vi "Generate_WayPoints_Hopping_IT_Surface.vi"(11 "Input Cluster":T2={"Scan Rate (um/s)"=15.0, "X Start"=15.0, "X End"=15.0, "Y Start"=15.0, "Y End"=15.0, " Z Start"=15.0, "HoppingDistance"=1.0, "V"=15.0, "Z End"=15.0, "Approach Rate Hopping (um/s)"=15.0, "Retrack Rate (um/s)"=15.0, "V 1"=15.0, "HoldTime IT/s"=15.0, "HoldTime Bulk Pre IT/s 2"=15.0, "HoldTime Bulk IT Post/s"=15.0, "V2"=0.0, "HoldTime IT 2/s"=15.0}) -> (0 "output cluster":T1, 3 "WaitTimeScaler":u64)   [LabVIEW 2023]
uses:
  TypeDefs/WayPointCluster.ctl
  TypeDefsControls/Time.ctl
  User_Vi/Settings.vi
panel:
  in  "WayPointCluster":T1
  out "Y  P":dbl
  out "X  P":dbl
  out "HoppingDistanceX":dbl
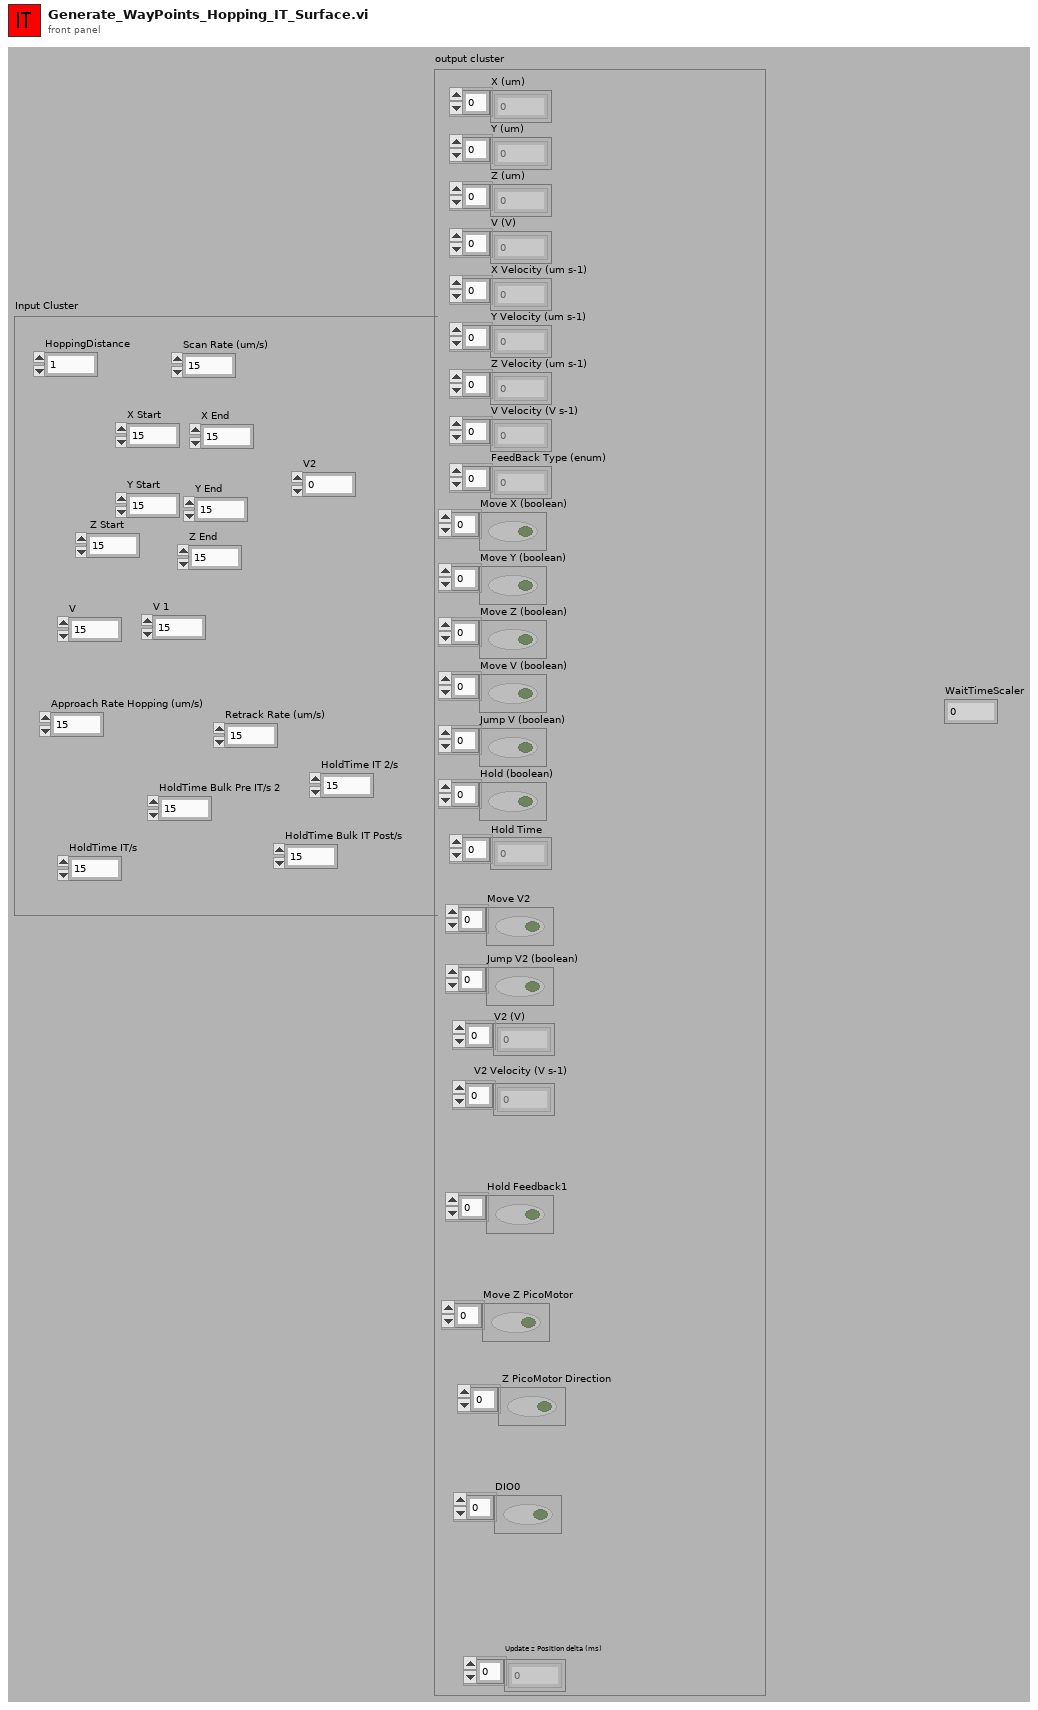
[diagram p1: front panel]
types:
  T1 = typedef "WayPointCluster.ctl" = cluster{"X (um)":dbl[], "Y (um)":dbl[], "Z (um)":dbl[], "V (V)":dbl[], "X Velocity (um s-1)":dbl[], "Y Velocity (um s-1)":dbl[], "Z Velocity (um s-1)":dbl[], "V Velocity (V s-1)":dbl[], "FeedBack Type (enum)":u16[], "Move X (boolean)":bool[], "Move Y (boolean)":bool[], "Move Z (boolean)":bool[], "Move V (boolean)":bool[], "Jump V (boolean)":bool[], "Hold (boolean)":bool[], "Hold Time":u32[], "V2 (V)":dbl[], "Move V2":bool[], "V2 Velocity (V s-1)":dbl[], "Jump V2 (boolean)":bool[], "Update z Position delta (ms)":i16[], "Hold Feedback1":bool[], "Move Z PicoMotor":bool[], " Z PicoMotor Direction":bool[], "DIO0":bool[]}
  T2 = cluster{"Scan Rate (um/s)":dbl, "X Start":dbl, "X End":dbl, "Y Start":dbl, "Y End":dbl, " Z Start":dbl, "HoppingDistance":dbl, "V":dbl, "Z End":dbl, "Approach Rate Hopping (um/s)":dbl, "Retrack Rate (um/s)":dbl, "V 1":dbl, "HoldTime IT/s":dbl, "HoldTime Bulk Pre IT/s 2":dbl, "HoldTime Bulk IT Post/s":dbl, "V2":dbl, "HoldTime IT 2/s":dbl}
  T3 = typedef "Time.ctl" = dbl
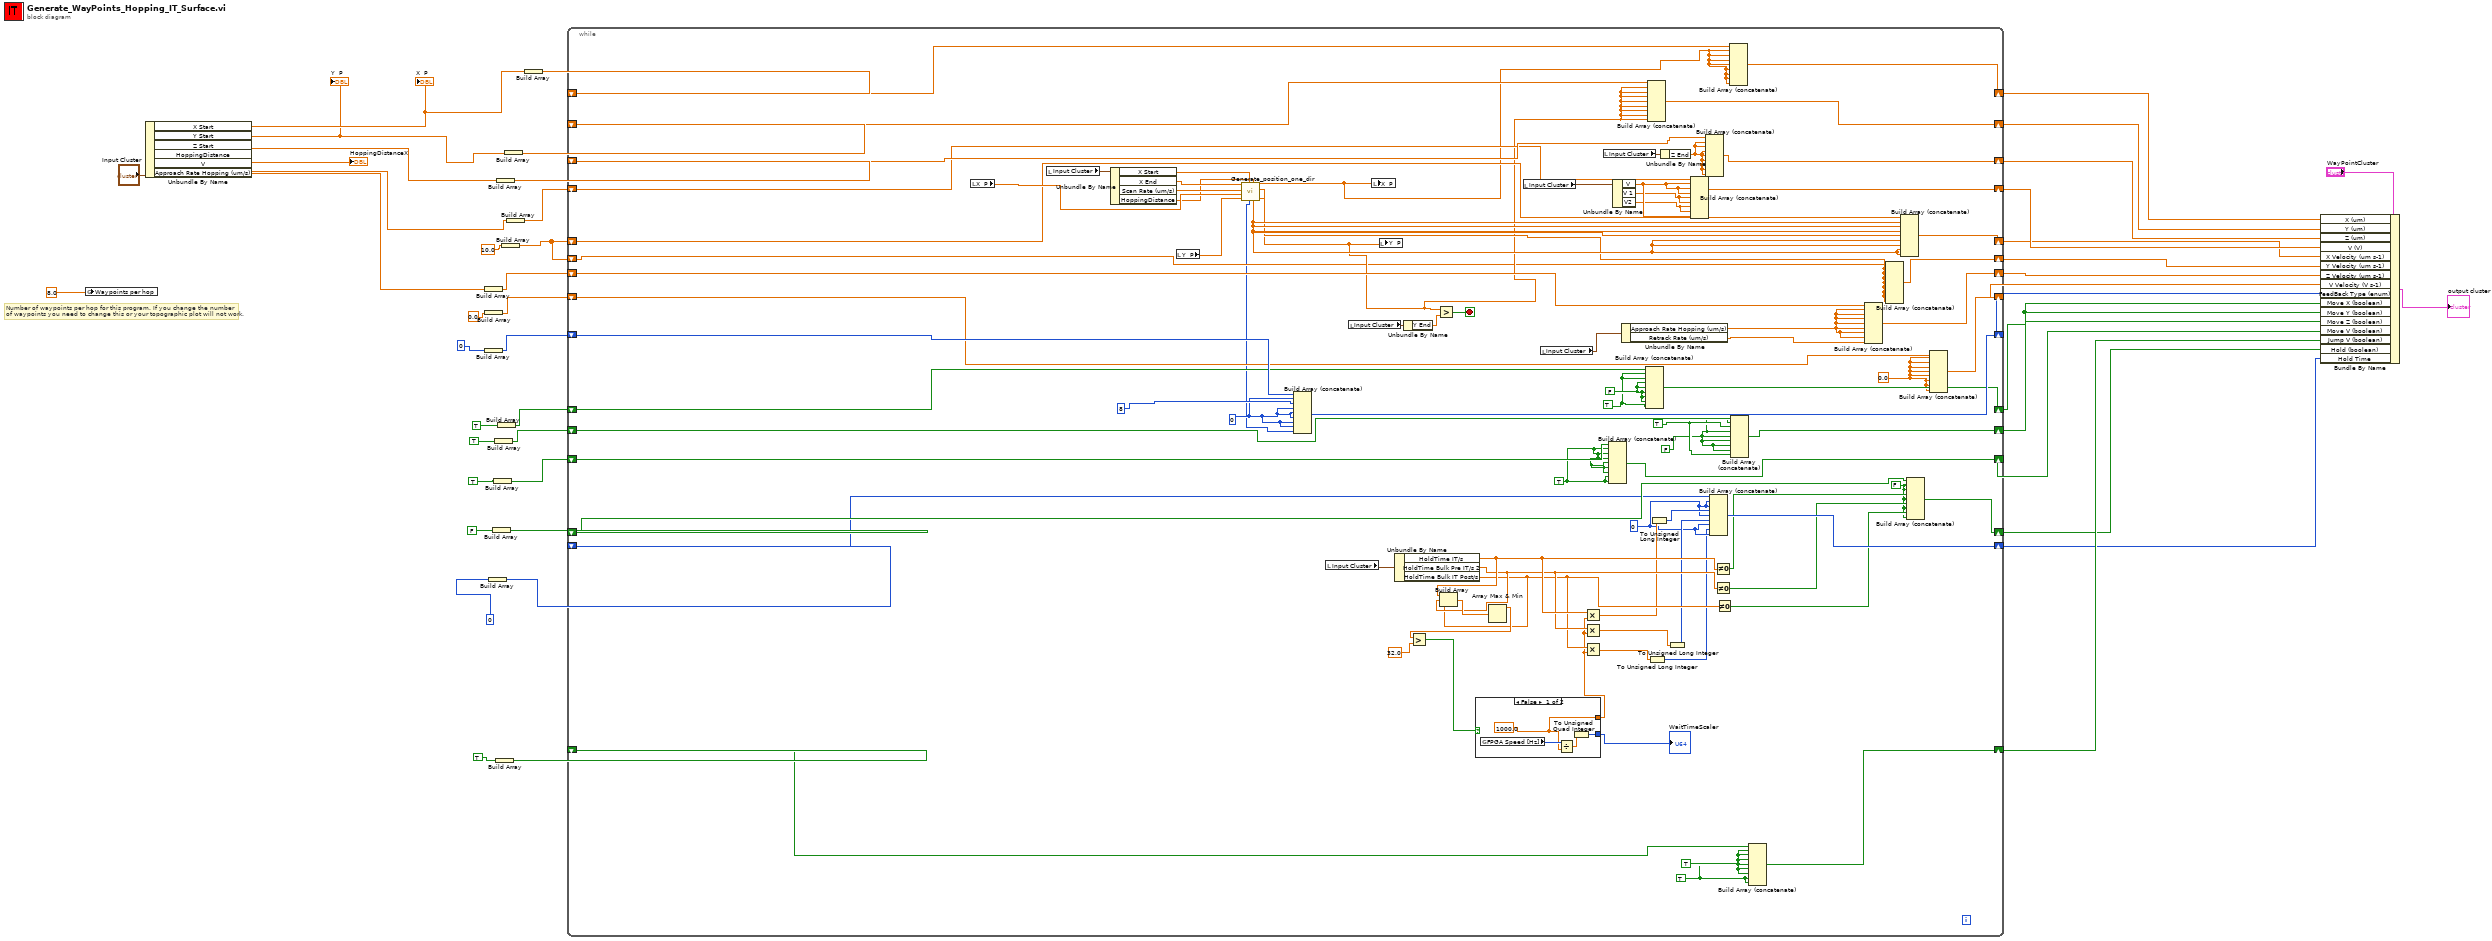
[diagram p0: block diagram]
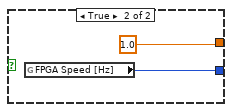
[diagram p2: hidden frame]
diagram:
  # "Number of waypoints per hop for this program. If you change the number\nof waypoints you need to change this or your topographic plot will not work."
  n1 = global write "Settings.vi" "Waypoints per hop"(8.0) -> ()
  n2 = Unbundle By Name("Input Cluster") -> ("X Start"=w31:dbl, "Y Start"=w30:dbl, "Z Start"=w32:dbl, "HoppingDistance"=→"HoppingDistanceX":dbl, "V"=w29:dbl, "Approach Rate Hopping (um/s)"=w17:dbl)
  "X  P" <- w31
  "Y  P" <- w30
  n3 = Build Array(w17) -> (w39:dbl[])
  n4 = Build Array(u64 0 ("element")) -> (w35:u64[])
  n5 = Build Array(0.0 ("element")) -> (w37:dbl[])
  n6 = Build Array(u64 0) -> (w4:u64[])
  n7 = Build Array(FALSE) -> (w20:bool[])
  n8 = Build Array(TRUE) -> (w24:bool[])
  n9 = Build Array(TRUE) -> (w28:bool[])
  n10 = Build Array(TRUE) -> (w26:bool[])
  n11 = Build Array(w32) -> (w43:dbl[])
  n12 = Build Array(TRUE) -> (w8:bool[])
  n13 = Build Array(10.0 ("element")) -> (w1:dbl[])
  n14 = Build Array(w30) -> (w45:dbl[])
  n15 = Build Array(w29) -> (w41:dbl[])
  n16 = Build Array(w31) -> (w47:dbl[])
  n17 = while {
    shift-right: [w125] -> w46
    shift-left: w47 -> [w100]
    shift-right: [w123] -> w44
    shift-left: w45 -> [w124]
    shift-right: [w121] -> w42
    shift-left: w43 -> [w122]
    shift-right: [w70] -> w40
    shift-left: w41 -> [w104]
    shift-right: [w120] -> w10
    shift-left: w1 -> [w90]
    shift-right: [w118] -> w38
    shift-left: w39 -> [w119]
    shift-right: [w116] -> w36
    shift-left: w37 -> [w117]
    shift-right: [w131] -> w34
    shift-left: w35 -> [w132]
    shift-right: [w114] -> w27
    shift-left: w28 -> [w115]
    shift-right: [w110] -> w13
    shift-left: w20 -> [w111]
    shift-right: [w81] -> w2
    shift-left: w4 -> [w109]
    shift-right: [w106] -> w25
    shift-left: w26 -> [w107]
    shift-right: [w112] -> w12
    shift-left: w24 -> [w113]
    shift-right: [w101] -> w7
    shift-left: w8 -> [w102]
    shift-right: [w91] -> w5
    shift-left: w1 -> [w69]
    stop <- w103 stop-if-true
    w50 = FALSE
    w55 = u32 0 ("element")
    w49 = TRUE
    w58 = FALSE
    w84 = 0.0 ("element")
    w105 = TRUE
    w83 = TRUE
    w82 = TRUE
    w64 = FALSE
    w65 = TRUE
    w67 = u64 0 ("element")
    n18 = local read "X  P"() -> (w96:dbl)
    n19 = local read "Input Cluster"() -> (w133:T2)
    n20 = Unbundle By Name(w133) -> ("X Start"=w95:dbl, "X End"=w94:dbl, "Scan Rate (um/s)"=w93:dbl, "HoppingDistance"=w92:dbl)
    n21 = local read "Y  P"() -> (w97:dbl)
    n22 = call "Generate_position_one_dir.vi"("HoppingDistance input"=w92, "X Start input"=w95, "Y P input"=w97, "X P input"=w96, "Scan Rate (um/s) input"=w93, "X end input"=w94) -> ("Y velocity output"=w85:dbl, "Y P output"=w72:dbl, "X P output"=w87:dbl, "X velocity output"=w86:dbl, "Feedback type retraction output"=w66:u64)  [unwired: 1 in]
    n23 = Build Array (concatenate)(w132, w67, u64 8, w67, w67, w67, w67, w67, w66) -> (w131:u64[])
    n24 = local read "Input Cluster"() -> (w108:T2)
    n25 = local read "Input Cluster"() -> (w128:T2)
    n26 = local write "X  P"(w87) -> ()
    n27 = local write "Y  P"(w72) -> ()
    n28 = Unbundle By Name(w108) -> ("HoldTime IT/s"=w80:dbl, "HoldTime Bulk Pre IT/s 2"=w79:dbl, "HoldTime Bulk IT Post/s"=w78:dbl)
    n29 = Unbundle By Name(w128) -> ("Y End"=w127:dbl)
    n30 = Greater?(x=w72, y=w127) -> (0:w103:bool)
    n31 = Build Array(w80, w79, w78) -> (w89:dbl[])
    n32 = Array Max & Min(array=w89) -> (max value=w88:dbl)  [unwired: 3 out]
    n33 = Greater?(x=w88, y=T3 32.0) -> (0:w98:bool)
    n34 = case shown="False" w98 {
      tunnel: [w135 w139] -> w73
      tunnel: [w134 1.0] -> w77
      frame False {
        w134 = 1000.0 ("y")
        n35 = global read "Settings.vi" "FPGA Speed [Hz]"() -> (w137:i64)
        n36 = Divide(x=w137, y=w134) -> (x/y=w136:dbl)
        n37 = To Unsigned Quad Integer(1:w136) -> (0:w135:u64)
      }
      frame True {
        n38 = global read "Settings.vi" "FPGA Speed [Hz]"() -> (w139:i64)
      }
    }
    "WaitTimeScaler" <- w73
    n39 = local read "Input Cluster"() -> (w129:T2)
    n40 = local read "Input Cluster"() -> (w126:T2)
    n41 = Multiply(x=w80, y=w77) -> (x*y=w76:dbl)
    n42 = Multiply(x=w79, y=w77) -> (x*y=w75:dbl)
    n43 = Multiply(x=w78, y=w77) -> (x*y=w74:dbl)
    n44 = local read "Input Cluster"() -> (w130:T2)
    n45 = Build Array (concatenate)(w113, w83, w83, w83, w83, w83, w83, w83, w83) -> (w112:bool[])
    n46 = Unbundle By Name(w129) -> ("V"=w63:dbl, "V 1"=w62:dbl, "V2"=w61:dbl)
    n47 = Unbundle By Name(w126) -> ("Approach Rate Hopping (um/s)"=w60:dbl, "Retrack Rate (um/s)"=w59:dbl)
    n48 = Build Array (concatenate)(w102, w49, w49, w58, w58, w58, w58, w58, w49) -> (w101:bool[])
    n49 = Build Array (concatenate)(w124, w72, w72, w72, w72, w72, w72, w72, w72) -> (w123:dbl[])
    n50 = To Unsigned Long Integer(number=w74) -> (unsigned 32bit integer=w54:u32)
    n51 = To Unsigned Long Integer(number=w76) -> (unsigned 32bit integer=w57:u32)
    n52 = Unbundle By Name(w130) -> ("Z End"=w71:dbl)
    n53 = To Unsigned Long Integer(number=w75) -> (unsigned 32bit integer=w56:u32)
    n54 = Build Array (concatenate)(w104, w63, w63, w63, w62, w62, w61, w61, w63) -> (w70:dbl[])
    n55 = Build Array (concatenate)(w122, w71, w71, w71, w71, w71, w71, w71, w71) -> (w121:dbl[])
    n56 = Build Array (concatenate)(w109, w55, w55, w57, w55, w56, w55, w54, w55) -> (w81:u64[])
    n57 = Not Equal To 0?(x=w80) -> (x != 0?=w53:bool)
    n58 = Not Equal To 0?(x=w79) -> (x != 0?=w52:bool)
    n59 = Not Equal To 0?(x=w78) -> (x != 0?=w51:bool)
    n60 = Build Array (concatenate)(w100, w87, w87, w87, w87, w87, w87, w87, w87) -> (w125:dbl[])
    n61 = Build Array (concatenate)(w115, w64, w65, w64, w64, w64, w64, w64, w65) -> (w114:bool[])
    n62 = Build Array (concatenate)(w107, w105, w105, w105, w82, w105, w105, w82, w82) -> (w106:bool[])
    n63 = Build Array (concatenate)(w119, w60, w60, w60, w60, w60, w60, w60, w59) -> (w118:dbl[])
    n64 = Build Array (concatenate)(w69, w85, w85, w85, w85, w85, w85, w85, w85) -> (w91:dbl[])
    n65 = Build Array (concatenate)(w90, w86, w86, w86, w86, w86, w86, w86, w86) -> (w120:dbl[])
    n66 = Build Array (concatenate)(w111, w50, w50, w53, w50, w52, w50, w51, w50) -> (w110:bool[])
    n67 = Build Array (concatenate)(w117, w84, w84, w84, w84, w84, w84, w84, w84) -> (w116:dbl[])
  }
  n68 = Bundle By Name(cluster="WayPointCluster", "X (um)"=w46, "Y (um)"=w44, "Z (um)"=w42, "V (V)"=w40, "X Velocity (um s-1)"=w10, "Y Velocity (um s-1)"=w5, "Z Velocity (um s-1)"=w38, "V Velocity (V s-1)"=w36, "FeedBack Type (enum)"=w34, "Move X (boolean)"=w7, "Move Y (boolean)"=w7, "Move Z (boolean)"=w27, "Move V (boolean)"=w12, "Jump V (boolean)"=w25, "Hold (boolean)"=w13, "Hold Time"=w2) -> (→"output cluster":T1)
